vi "GCode Parser.vi"(8 "error in (no error)":errorcluster, 9 "Comment char":string[](array[string])=[";", "("], 10 "Search Tokens":string[](array[string])=["G", "M", "X", "Y", "Z", "I", "J", "S", "F", "E", "N"], 11 "String in":string) -> (0 "error out":errorcluster, 3 "Command Array":T1[](array[typedef]))   [LabVIEW 2017]
doc: "This GCode parser extracts the GCode commands into an \"Command Array\". Command Array contains the parameters for each command."
uses:
  GCode Command Cluster.ctl
panel:
  out "Array (for debug)":string[][](array[string])
  # "USE EOL as end."
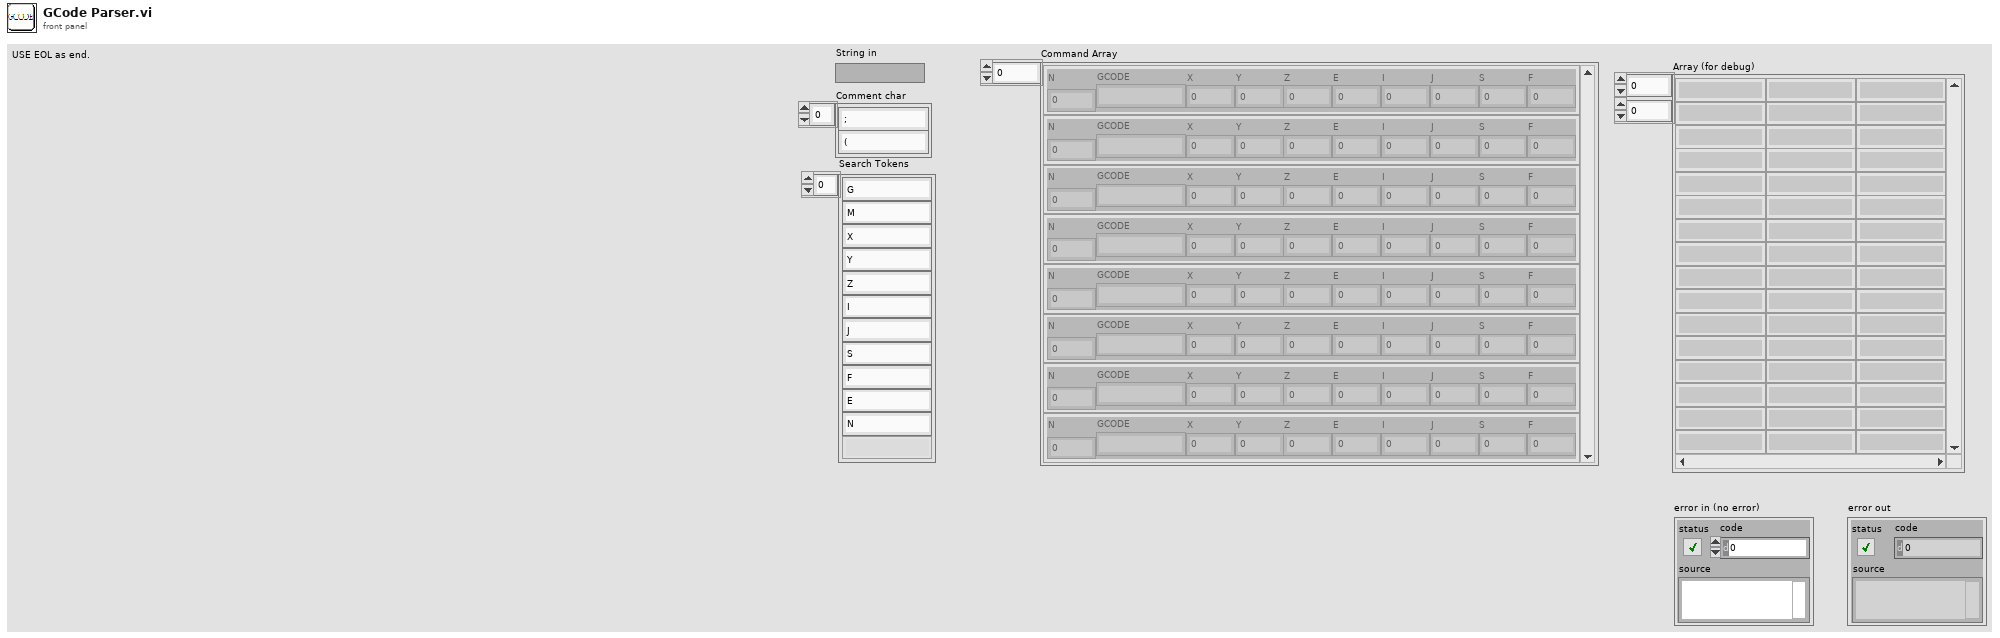
[diagram p1: front panel]
types:
  T1 = typedef "GCode Command Cluster.ctl" = cluster{"N":dbl, "GCODE":string, "X":dbl, "Y":dbl, "Z":dbl, "E":dbl, "I":dbl, "J":dbl, "S":dbl, "F":dbl}
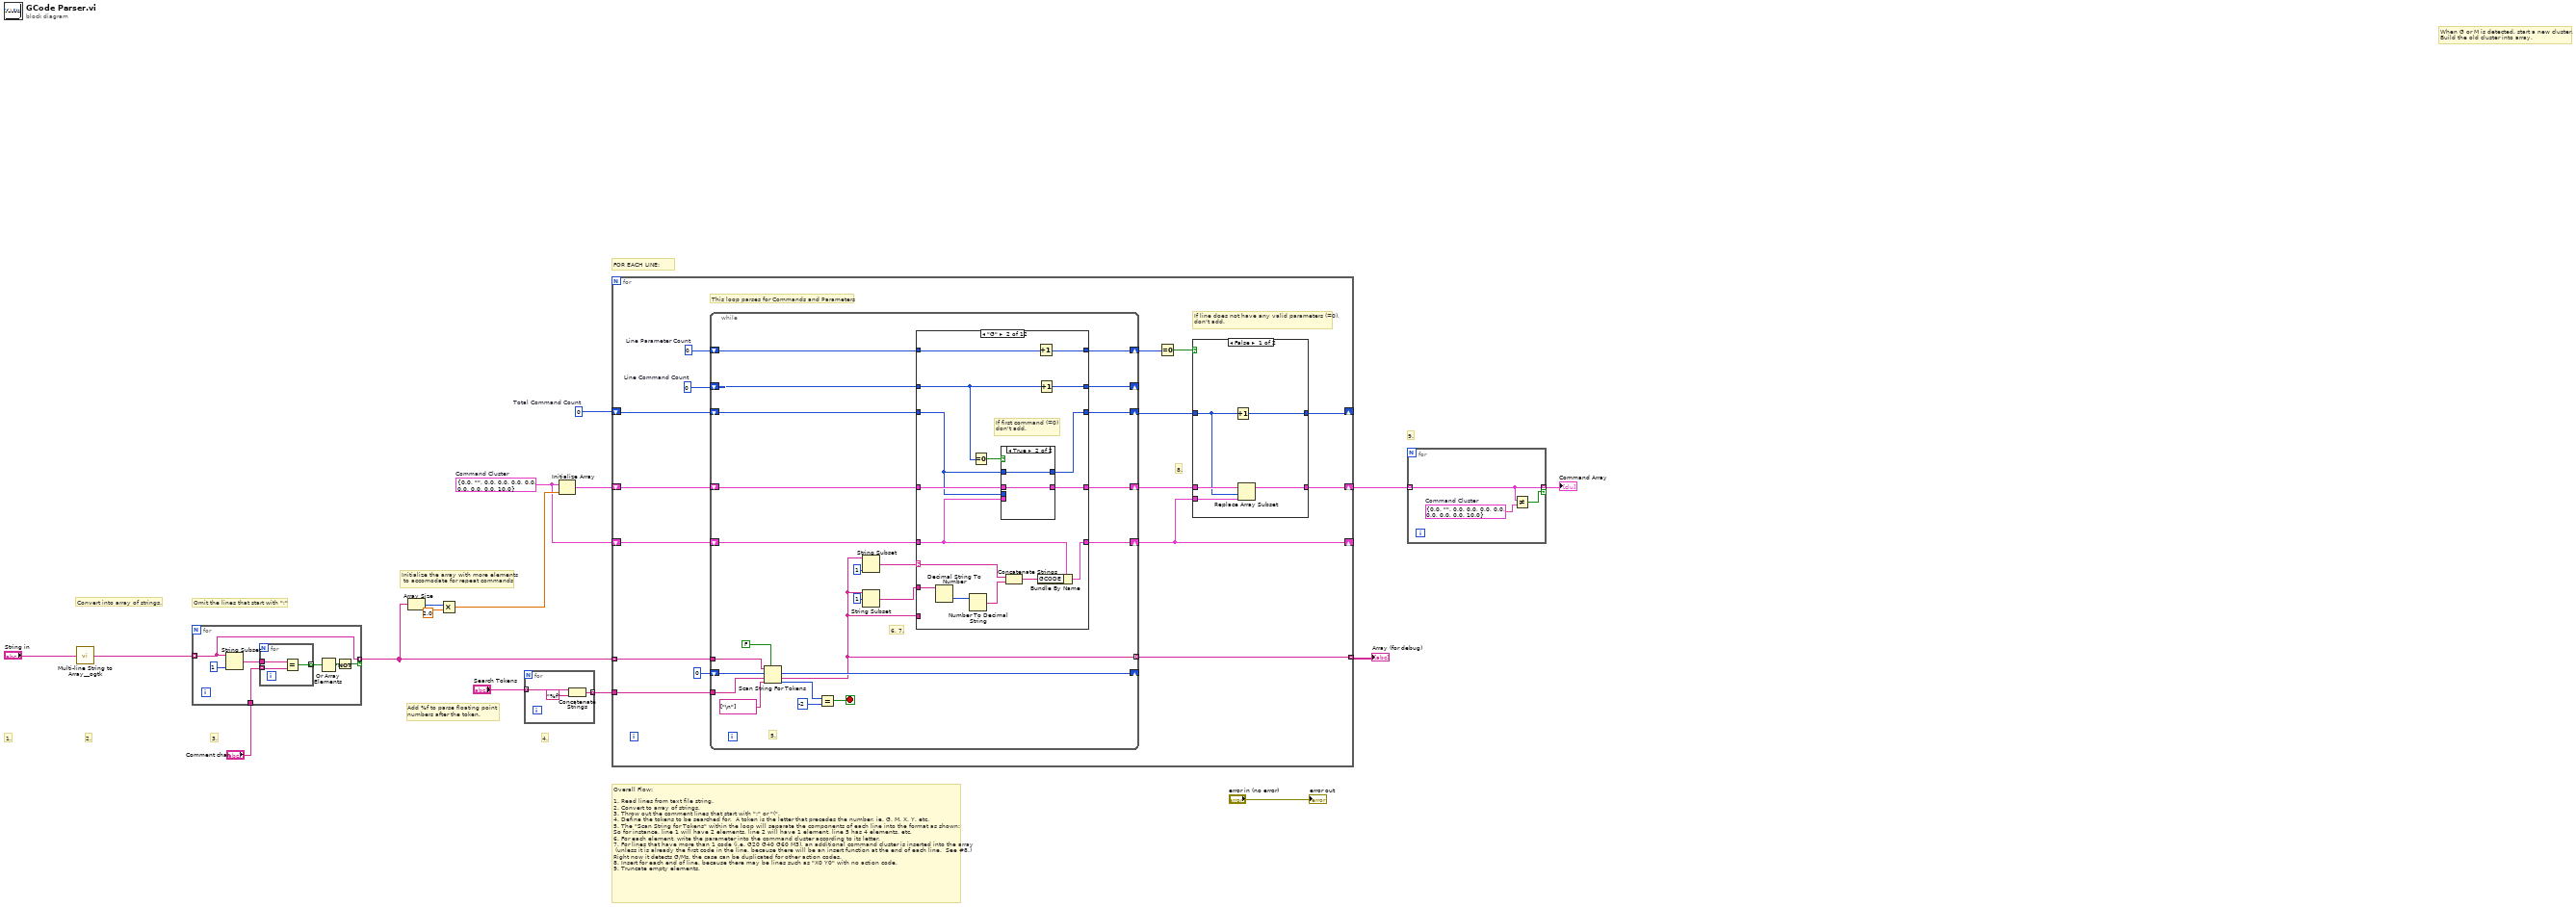
[diagram p0: block diagram]
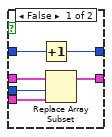
[diagram p4: hidden frame]
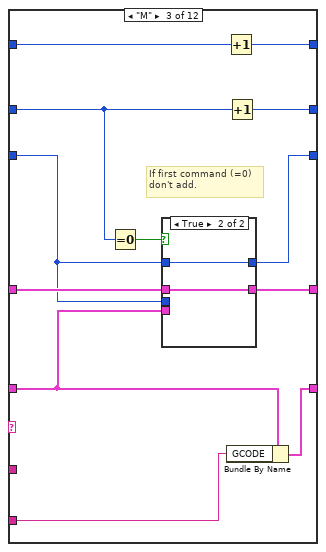
[diagram p5: hidden frame]
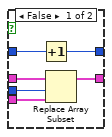
[diagram p6: hidden frame]
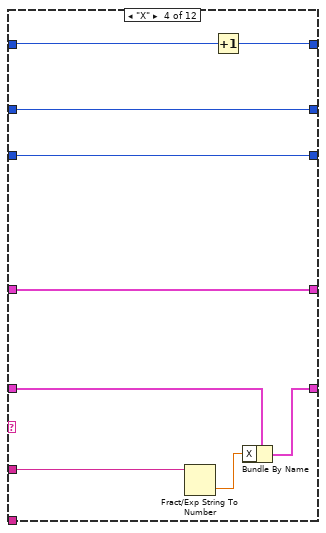
[diagram p7: hidden frame]
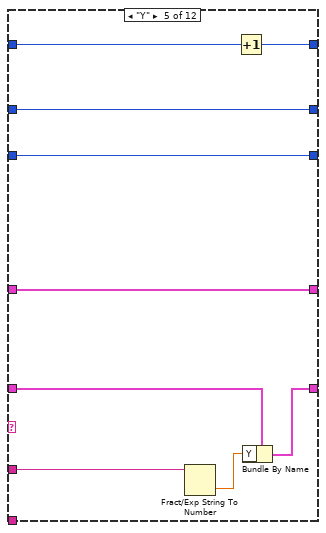
[diagram p8: hidden frame]
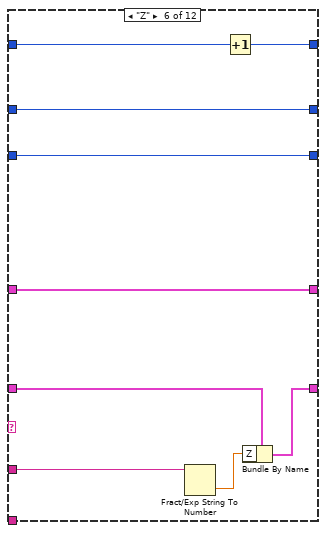
[diagram p9: hidden frame]
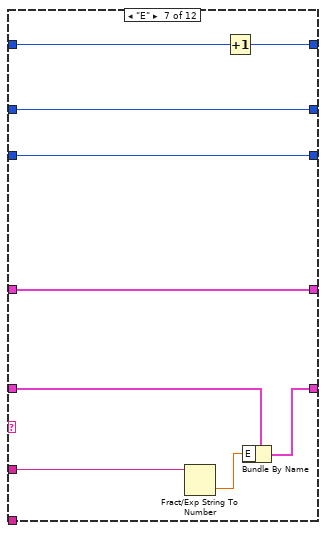
[diagram p10: hidden frame]
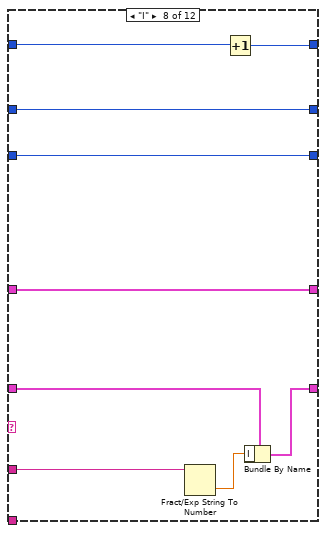
[diagram p11: hidden frame]
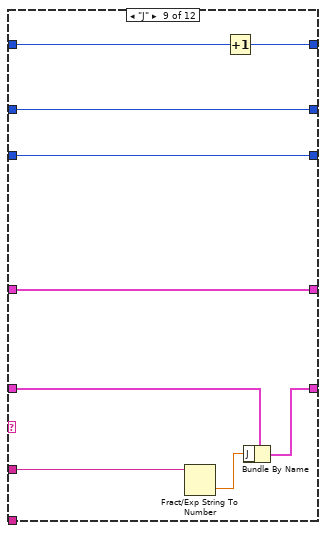
[diagram p12: hidden frame]
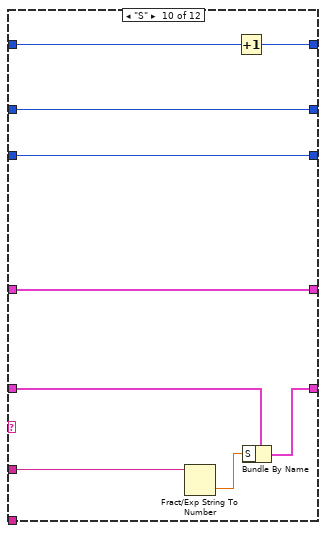
[diagram p13: hidden frame]
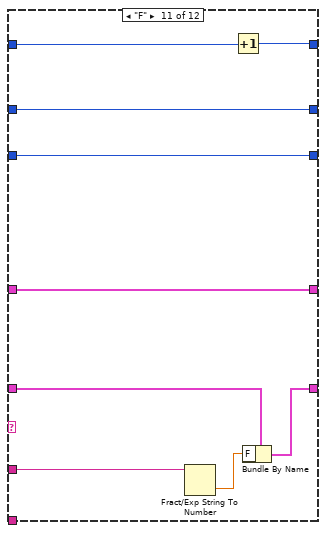
[diagram p14: hidden frame]
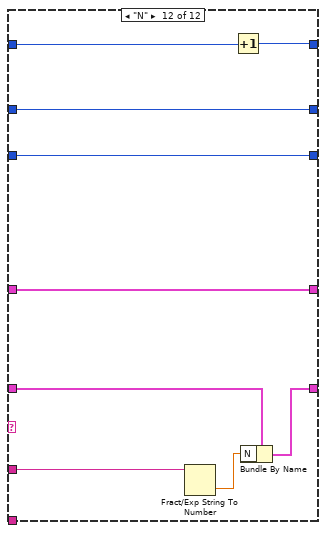
[diagram p15: hidden frame]
diagram:
  w7 = T1 {"N"=0.0, "GCODE"="", "X"=0.0, "Y"=0.0, "Z"=0.0, "E"=0.0, "I"=0.0, "J"=0.0, "S"=0.0, "F"=10.0}  # Command Cluster
  w12 = 0  # Total Command Count
  # "9."
  # "Initialize the array with more elements\n to accomodate for repeat commands"
  # "Convert into array of strings."
  # "4."
  # "3."
  # "2."
  # "1."
  # "Overall Flow:\n\n1.\tRead lines from text file string.\n2.\tConvert to array of strings.\n3.\tThrow out the comment lines that start with \";\" or \"(\". \n4.\tDefine the tokens to be searched for.  A token is the letter that precedes the number, ie. G, M, X, Y, etc.\n5.\tThe \"Scan String for Tokens\" within the loop will separate the components of each line into the format as shown: \nSo for instance, line 1 will have 2 elements, line 2 will have 1 element, line 5 has 4 elements, etc.\n6.\tFor each element, write the parameter into the command cluster according to its letter.\n7.\tFor lines that have more than 1 code (i.e. G20 G40 G60 M3), an additional command cluster is inserted into the array\n (unless it is already the first code in the line, because there will be an insert function at the end of each line.  See #8.)  \nRight now it detects G/Ms, the case can be duplicated for other action codes.\n8.\tInsert for each end of line, because there may be lines such as \"X0 Y0\" with no action code.\n9. Truncate empty elements."
  # "Add %f to parse floating point \nnumbers after the token."
  # "FOR EACH LINE:"
  # "Omit the lines that start with \";\""
  # "When G or M is detected, start a new cluster.\nBuild the old cluster into array."
  n1 = call "Multi-line String to Array__ogtk.vi"("string"="String in") -> ("lines"=w16:string[])
  n2 = for {
    tunnel: w16 -> [w21] mode=indexing
    tunnel: [w21] -> w11 mode=indexing if=w22
    tunnel: "Comment char" -> [w20]
    n3 = String Subset(string=w21, length (rest)=1 ("length (rest)")) -> (substring=w19:string)  [unwired: 1 in]
    n4 = for {
      tunnel: w20 -> [w25] mode=indexing
      tunnel: w19 -> [w26]
      tunnel: [w24] -> w18 mode=indexing
      n5 = Equal?(x=w26, y=w25) -> (x = y?=w24:bool)
    }
    n6 = Or Array Elements(Boolean array=w18) -> (logical OR=w17:bool)
    n7 = Not(x=w17) -> (.not. x?=w22:bool)
  }
  n8 = Array Size(array=w11) -> (size(s)=w10:i32)
  n9 = Multiply(x=w10, y=2.0) -> (x*y=w8:dbl)
  n10 = for {
    tunnel: "Search Tokens" -> [w29] mode=indexing
    tunnel: [w27] -> w14 mode=indexing
    n11 = Concatenate Strings(w29, "%f" ("string")) -> (w27:string)
  }
  n12 = Initialize Array "Initialize Array"(w7, w8) -> (w13:T1[])
  n13 = for {
    tunnel: w11 -> [w44] mode=indexing
    shift-right: [w35] -> _
    shift-left: w7 -> [w43]
    tunnel: w14 -> [w42]
    shift-right: [w30] -> w5
    shift-left: w13 -> [w41]
    shift-right: [w36] -> _
    shift-left: w12 -> [w39]
    tunnel: [w31] -> w6 mode=indexing
    w33 = 0  # Line Parameter Count
    w40 = 0  # Line Command Count
    # "8."
    # "If line does not have any valid parameters (=0),\ndon't add."
    # "This loop parses for Commands and Parameters"
    n14 = while {
      tunnel: w42 -> [w76]
      tunnel: w44 -> [w71]
      shift-right: [w74] -> _
      shift-left: 0 ("offset past token") -> [w75]
      shift-right: [w66] -> w35
      shift-left: w43 -> [w60]
      shift-right: [w61] -> w38
      shift-left: w41 -> [w57]
      shift-right: [w62] -> _
      shift-left: w40 -> [w63]
      shift-right: [w59] -> w37
      shift-left: w39 -> [w58]
      shift-right: [w54] -> w32
      shift-left: w33 -> [w55]
      tunnel: [w53] -> w31 mode=indexing
      stop <- w65 stop-if-true
      # "6, 7."
      # "5."
      n15 = Scan String For Tokens(5:FALSE ("allow empty tokens? (F)"), 6:string[] ["\n"] ("delimiters (\\s,\\t,\\r,\\n)"), 7:w76, 8:w75, 9:w71) -> (0:w72:i32, 1:w53:string, 2:w74:i32)  [unwired: 1 in, 1 out]
      n16 = Equal?(x=w72, y=-2) -> (x = y?=w65:bool)
      n17 = String Subset(string=w53, length (rest)=1 ("length (rest)")) -> (substring=w68:string)  [unwired: 1 in]
      n18 = String Subset(string=w53, offset (0)=1) -> (substring=w67:string)  [unwired: 1 in]
      n19 = case shown="\"G\"" w68 {
        selector: w68 -> [_ w83 _ _ _ _ _ _ _ _ _ _]
        tunnel: [w81 w97 w117 w134 w143 w152 w161 w170 w179 w188 w197 w206] -> w66
        tunnel: w67 -> [_ w86 _ w132 w141 w150 w159 w168 w177 w186 w195 w204]
        tunnel: w60 -> [w81 w93 w112 w131 w140 w149 w158 w167 w176 w185 w194 w203]
        tunnel: w53 -> [_ _ w116 _ _ _ _ _ _ _ _ _]
        tunnel: w63 -> [w80 w94 w113 w130 w139 w148 w157 w166 w175 w184 w193 w202]
        tunnel: [w80 w92 w111 w130 w139 w148 w157 w166 w175 w184 w193 w202] -> w62
        tunnel: w57 -> [w79 w95 w114 w129 w138 w147 w156 w165 w174 w183 w192 w201]
        tunnel: [w79 w96 w115 w129 w138 w147 w156 w165 w174 w183 w192 w201] -> w61
        tunnel: w58 -> [w78 w91 w110 w128 w137 w146 w155 w164 w173 w182 w191 w200]
        tunnel: [w78 w90 w109 w128 w137 w146 w155 w164 w173 w182 w191 w200] -> w59
        tunnel: w55 -> [w77 w88 w107 w127 w136 w145 w154 w163 w172 w181 w190 w199]
        tunnel: [w77 w87 w106 w126 w135 w144 w153 w162 w171 w180 w189 w198] -> w54
        frame Default {
        }
        frame "G" {
          # "If first command (=0)\ndon't add."
          n20 = Decimal String To Number(string=w86) -> (number=w85:i32)  [unwired: 2 in, 1 out]
          n21 = Number To Decimal String(number=w85) -> (decimal integer string=w84:string)  [unwired: 1 in]
          n22 = Equal To 0?(x=w94) -> (x = 0?=w89:bool)
          n23 = case shown="True" w89 {
            tunnel: w93 -> [w103 _]
            tunnel: [w101 w105] -> w96
            tunnel: w95 -> [w102 w105]
            tunnel: w91 -> [w100 _]
            tunnel: w91 -> [w99 w104]
            tunnel: [w98 w104] -> w90
            frame False {
              n24 = Increment(x=w99) -> (x+1=w98:i32)
              n25 = Replace Array Subset(array=w102, new element=w103, index=w100) -> (w101:T1[])
            }
            frame True {
            }
          }
          n26 = Concatenate Strings(w83, w84) -> (w82:string)
          n27 = Increment(x=w88) -> (x+1=w87:i32)
          n28 = Increment(x=w94) -> (x+1=w92:i32)
          n29 = Bundle By Name(cluster=w93, "GCODE"=w82) -> (w97:T1)
        }
        frame "M" {
          # "If first command (=0)\ndon't add."
          n30 = Equal To 0?(x=w113) -> (x = 0?=w108:bool)
          n31 = case shown="True" w108 {
            tunnel: w112 -> [w123 _]
            tunnel: [w121 w125] -> w115
            tunnel: w114 -> [w122 w125]
            tunnel: w110 -> [w120 _]
            tunnel: w110 -> [w119 w124]
            tunnel: [w118 w124] -> w109
            frame False {
              n32 = Increment(x=w119) -> (x+1=w118:i32)
              n33 = Replace Array Subset(array=w122, new element=w123, index=w120) -> (w121:T1[])
            }
            frame True {
            }
          }
          n34 = Increment(x=w107) -> (x+1=w106:i32)
          n35 = Increment(x=w113) -> (x+1=w111:i32)
          n36 = Bundle By Name(cluster=w112, "GCODE"=w116) -> (w117:T1)
        }
        frame "X" {
          n37 = Fract/Exp String To Number(string=w132) -> (number=w133:dbl)  [unwired: 3 in, 1 out]
          n38 = Increment(x=w127) -> (x+1=w126:i32)
          n39 = Bundle By Name(cluster=w131, "X"=w133) -> (w134:T1)
        }
        frame "Y" {
          n40 = Fract/Exp String To Number(string=w141) -> (number=w142:dbl)  [unwired: 3 in, 1 out]
          n41 = Increment(x=w136) -> (x+1=w135:i32)
          n42 = Bundle By Name(cluster=w140, "Y"=w142) -> (w143:T1)
        }
        frame "Z" {
          n43 = Fract/Exp String To Number(string=w150) -> (number=w151:dbl)  [unwired: 3 in, 1 out]
          n44 = Increment(x=w145) -> (x+1=w144:i32)
          n45 = Bundle By Name(cluster=w149, "Z"=w151) -> (w152:T1)
        }
        frame "E" {
          n46 = Fract/Exp String To Number(string=w159) -> (number=w160:dbl)  [unwired: 3 in, 1 out]
          n47 = Increment(x=w154) -> (x+1=w153:i32)
          n48 = Bundle By Name(cluster=w158, "E"=w160) -> (w161:T1)
        }
        frame "I" {
          n49 = Fract/Exp String To Number(string=w168) -> (number=w169:dbl)  [unwired: 3 in, 1 out]
          n50 = Increment(x=w163) -> (x+1=w162:i32)
          n51 = Bundle By Name(cluster=w167, "I"=w169) -> (w170:T1)
        }
        frame "J" {
          n52 = Fract/Exp String To Number(string=w177) -> (number=w178:dbl)  [unwired: 3 in, 1 out]
          n53 = Increment(x=w172) -> (x+1=w171:i32)
          n54 = Bundle By Name(cluster=w176, "J"=w178) -> (w179:T1)
        }
        frame "S" {
          n55 = Fract/Exp String To Number(string=w186) -> (number=w187:dbl)  [unwired: 3 in, 1 out]
          n56 = Increment(x=w181) -> (x+1=w180:i32)
          n57 = Bundle By Name(cluster=w185, "S"=w187) -> (w188:T1)
        }
        frame "F" {
          n58 = Fract/Exp String To Number(string=w195) -> (number=w196:dbl)  [unwired: 3 in, 1 out]
          n59 = Increment(x=w190) -> (x+1=w189:i32)
          n60 = Bundle By Name(cluster=w194, "F"=w196) -> (w197:T1)
        }
        frame "N" {
          n61 = Fract/Exp String To Number(string=w204) -> (number=w205:dbl)  [unwired: 3 in, 1 out]
          n62 = Increment(x=w199) -> (x+1=w198:i32)
          n63 = Bundle By Name(cluster=w203, "N"=w205) -> (w206:T1)
        }
      }
    }
    n64 = Equal To 0?(x=w32) -> (x = 0?=w34:bool)
    n65 = case shown="False" w34 {
      tunnel: w38 -> [w50 w51]
      tunnel: w35 -> [w49 _]
      tunnel: [w48 w52] -> w36
      tunnel: w37 -> [w47 w52]
      tunnel: [w46 w51] -> w30
      frame False {
        n66 = Increment(x=w47) -> (x+1=w48:i32)
        n67 = Replace Array Subset "Replace Array Subset"(array=w50, new element=w49, index=w47) -> (w46:T1[])
      }
      frame True {
      }
    }
  }
  "Array (for debug)" <- w6
  n68 = for {
    tunnel: w5 -> [w208] mode=indexing
    tunnel: [w208] -> w4 mode=indexing if=w207
    w209 = T1 {"N"=0.0, "GCODE"="", "X"=0.0, "Y"=0.0, "Z"=0.0, "E"=0.0, "I"=0.0, "J"=0.0, "S"=0.0, "F"=10.0}  # Command Cluster
    n69 = Not Equal?(x=w208, y=w209) -> (x != y?=w207:bool)
  }
  "Command Array" <- w4
  "error out" <- "error in (no error)"
